vi "Instrument jsObject.vi"(8 "error in (no error)":errorcluster, 9 "Instrument Record (empty)":T1, 10 "Instrument Object Name (\"\")":string, 11 "Previous String (\"\")":string) -> (0 "error out":errorcluster, 2 "Instrument jsObject":string, 3 "Instrument Definition":string)   [LabVIEW 2011]
uses:
  Instrument Record.ctl
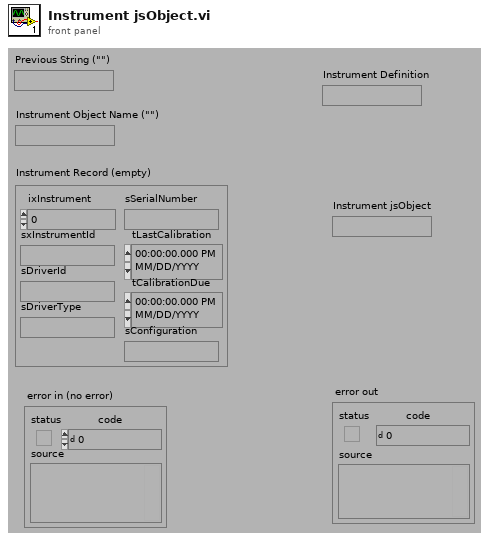
[diagram p1: front panel]
types:
  T1 = typedef "Instrument Record.ctl" = cluster{"ixInstrument":i32, "sxInstrumentId":string, "sDriverId":string, "sDriverType":string, "sSerialNumber":string, "tLastCalibration":timestamp, "tCalibrationDue":timestamp, "sConfiguration":string}
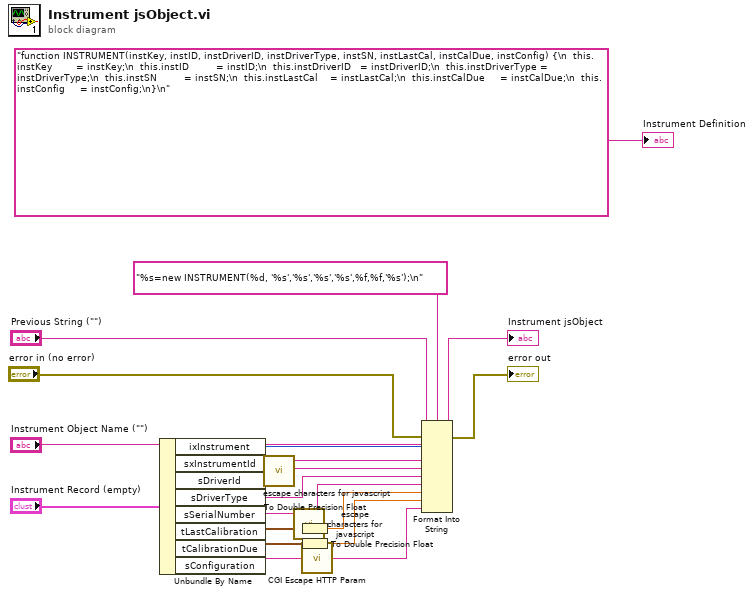
[diagram p0: block diagram]
diagram:
  n1 = Unbundle By Name("Instrument Record (empty)") -> ("ixInstrument"=w10:i32, "sxInstrumentId"=w9:string, "sDriverId"=w20:string, "sDriverType"=w19:string, "sSerialNumber"=w7:string, "tLastCalibration"=w4:timestamp, "tCalibrationDue"=w2:timestamp, "sConfiguration"=w18:string)
  n2 = call "escape characters for javascript.vi"("String (\"\")"=w9) -> ("escaped String"=w8:string)  [unwired: 4 out]
  n3 = call "escape characters for javascript.vi"("String (\"\")"=w7) -> ("escaped String"=w6:string)  [unwired: 4 out]
  n4 = To Double Precision Float(number=w4) -> (double precision float=w3:dbl)
  n5 = To Double Precision Float(number=w2) -> (double precision float=w1:dbl)
  n6 = call "CGI Escape HTTP Param.vi"("string"=w18) -> ("url-encoded string"=w17:string)
  n7 = Format Into String(format string="%s=new INSTRUMENT(%d, '%s','%s','%s','%s',%f,%f,'%s');\n", initial string="Previous String (\"\")", error in="error in (no error)", "Instrument Object Name (\"\")", w10, w8, w20, w19, w6, w3, w1, w17) -> (resulting string=→"Instrument jsObject":string, error out=→"error out":errorcluster)
  "Instrument Definition" <- "function INSTRUMENT(instKey, instID, instDriverID, instDriverType, instSN, instLastCal, instCalDue, instConfig) {\n  this.instKey        = instKey;\n  this.instID         = instID;\n  this.instDriverID   = instDriverID;\n  this.instDriverType = instDriverType;\n  this.instSN         = instSN;\n  this.instLastCal    = instLastCal;\n  this.instCalDue     = instCalDue;\n  this.instConfig     = instConfig;\n}\n"
